vi "Test MQTT-3.9.3-2.vi"(8 "error in (no error)":errorcluster) -> (0 "error out":errorcluster)   [LabVIEW 2013]
uses:
  source/Control Packets/SUBACK/Subscription Success Code.ctl
  source/Control Packets/ControlPacket/QualityOfService -- enum.ctl
  <vilib>/addons/_JKI Toolkits/Caraya/classes/Test/Test.lvclass
  source/Control Packets/ControlPacket/ControlPacket.lvclass
  source/Control Packets/SUBACK/SUBACK.lvclass
  <vilib>/addons/_JKI Toolkits/Caraya/classes/Assert/Assert.lvclass
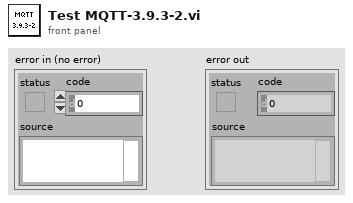
[diagram p1: front panel]
types:
  T1 = typedef "SUBACK.lvclass/Subscription Success Code.ctl" = cluster{"Subscription Failure":bool, "QoS":T2}
  T2 = typedef "ControlPacket.lvclass/QualityOfService -- enum.ctl" = enum16{"0 (At Most Once)", "1 (At Least Once)", "2 (Exactly Once)"}
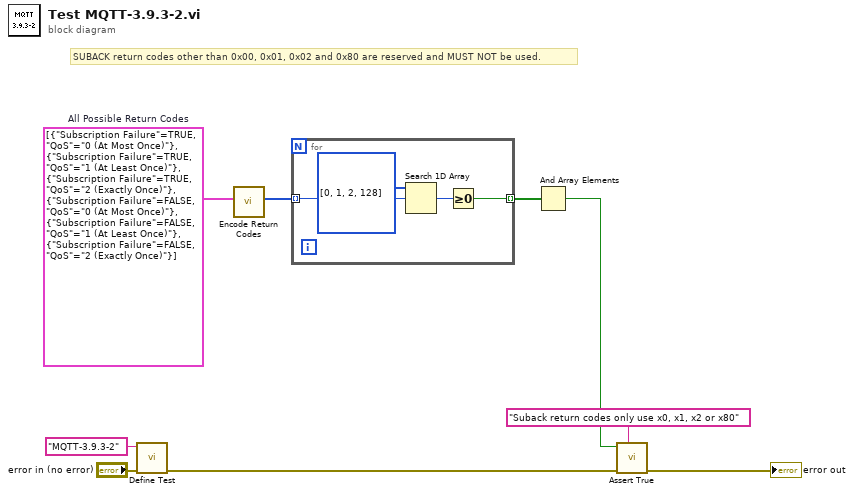
[diagram p0: block diagram]
diagram:
  w6 = T1[] [{"Subscription Failure"=TRUE, "QoS"=enum."0 (At Most Once)"}, {"Subscription Failure"=TRUE, "QoS"=enum."1 (At Least Once)"}, {"Subscription Failure"=TRUE, "QoS"=enum."2 (Exactly Once)"}, {"Subscription Failure"=FALSE, "QoS"=enum."0 (At Most Once)"}, {"Subscription Failure"=FALSE, "QoS"=enum."1 (At Least Once)"}, {"Subscription Failure"=FALSE, "QoS"=enum."2 (Exactly Once)"}]  # All Possible Return Codes
  # "SUBACK return codes other than 0x00, 0x01, 0x02 and 0x80 are reserved and MUST NOT be used."
  n1 = call <vilib>:"Define Test.vi"("error in (no error)"="error in (no error)", "Label (VI Title)"="MQTT-3.9.3-2") -> ("error out"=w2:errorcluster)  [unwired: 9 in]
  n2 = call "Encode Return Codes.vi"("Subscription Success"=w6) -> ("Return Codes"=w5:u8[])  [unwired: 10 in]
  n3 = for {
    tunnel: w5 -> [w13] mode=indexing
    tunnel: [w10] -> w4 mode=indexing
    n4 = Search 1D Array(1D array=u8[] [0, 1, 2, 128], element=w13) -> (index of element=w11:i32)  [unwired: 1 in]
    n5 = Greater Or Equal To 0?(x=w11) -> (x >= 0?=w10:bool)
  }
  n6 = And Array Elements(Boolean array=w4) -> (logical AND=w3:bool)
  n7 = call <vilib>:"Assert True.vi"("Label"="Suback return codes only use x0, x1, x2 or x80", "error in (no error)"=w2, "True?"=w3) -> ("error out"=→"error out":errorcluster)  [unwired: 8 in]
